vi "sub_flood-fill.vi"(10 "occupancy_map":T1, 11 "center_point":cluster{"center x":i32, "center y":i32}) -> ()   [LabVIEW 2019]
uses:
  <vilib>/Analysis/Matrix/Datatypes/RealMatrix.ctl
  <vilib>/Analysis/Matrix/NI_Matrix.lvlib
panel:
  out "sy":i32
  out "sx":i32
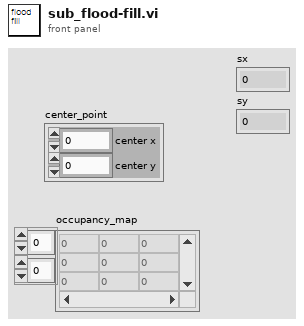
[diagram p1: front panel]
types:
  T1 = typedef "NI_Matrix.lvlib/RealMatrix.ctl" = dbl[][]
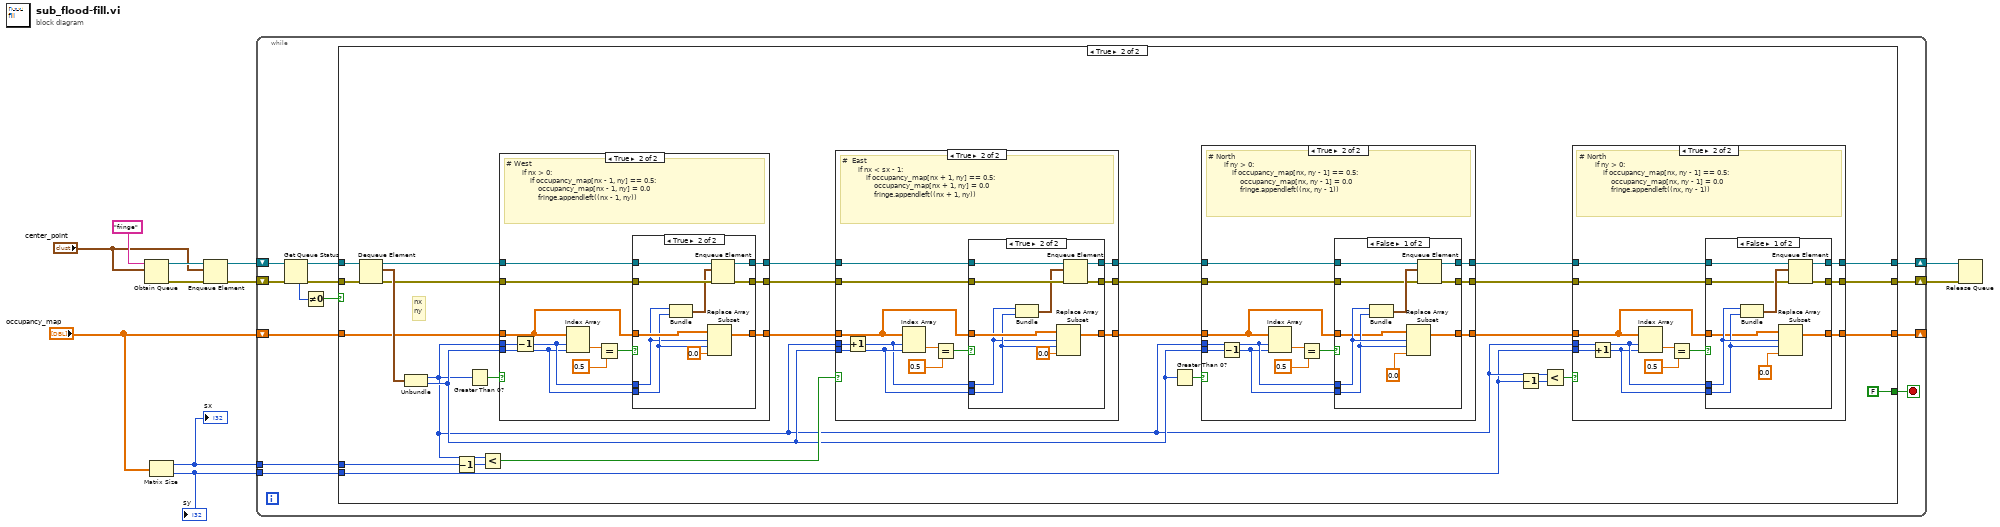
[diagram p0: block diagram]
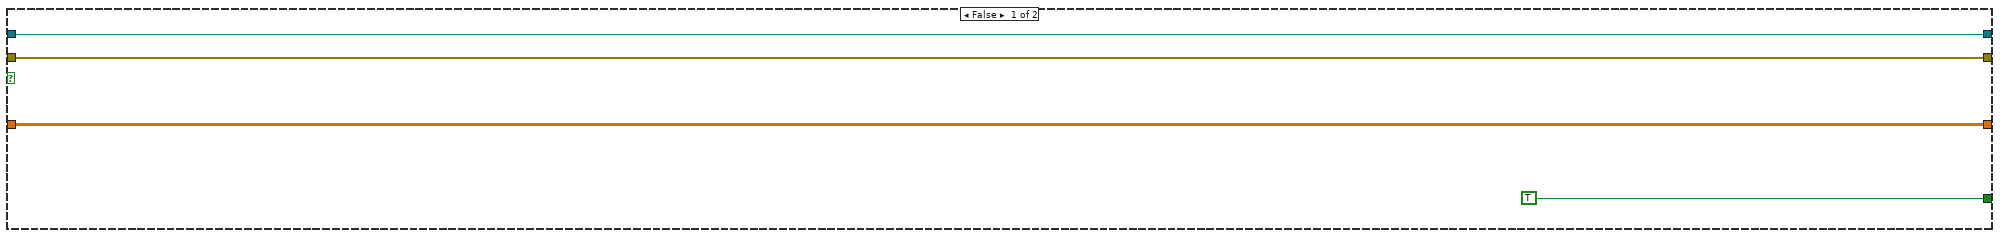
[diagram p2: hidden frame]
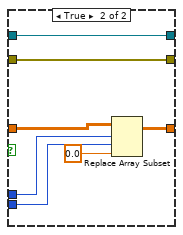
[diagram p4: hidden frame]
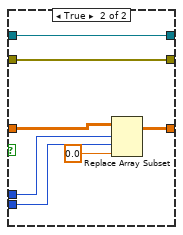
[diagram p6: hidden frame]
diagram:
  n1 = Obtain Queue(name (unnamed)="fringe", element data type="center_point") -> (queue out=w9:refnum<queue>, error out=w10:errorcluster)  [unwired: 3 in, 1 out]
  n2 = Matrix Size(0:"occupancy_map") -> (1:w2:i32, 2:w1:i32)
  "sx" <- w2
  "sy" <- w1
  n3 = Enqueue Element(queue=w9, element="center_point", error in (no error)=w10) -> (queue out=w6:refnum<queue>, error out=w7:errorcluster)  [unwired: 1 in, 1 out]
  n4 = while {
    shift-right: [w17] -> w5
    shift-left: w6 -> [w23]
    shift-right: [w16] -> w4
    shift-left: w7 -> [w24]
    shift-right: [w14] -> _
    shift-left: "occupancy_map" -> [w15]
    tunnel: w2 -> [w13]
    tunnel: w1 -> [w12]
    stop <- w20 stop-if-true
    n5 = Get Queue Status(queue=w23, error in (no error)=w24) -> (queue out=w18:refnum<queue>, error out=w19:errorcluster, # elements in queue=w22:i32)  [unwired: 1 in, 5 out]
    n6 = Not Equal To 0?(x=w22) -> (x != 0?=w21:bool)
    n7 = case shown="True" w21 {
      tunnel: [TRUE FALSE] -> w20
      tunnel: w19 -> [w26 w56]
      tunnel: w18 -> [w27 w55]
      tunnel: [w27 w36] -> w17
      tunnel: [w26 w35] -> w16
      tunnel: w15 -> [w25 w52]
      tunnel: [w25 w33] -> w14
      tunnel: w13 -> [_ w49]
      tunnel: w12 -> [_ w29]
      frame False {
      }
      frame True {
        # "nx\nny"
        n8 = Dequeue Element(queue=w55, error in (no error)=w56) -> (queue out=w44:refnum<queue>, element=w54:cluster{"center x":i32, "center y":i32}, error out=w41:errorcluster)  [unwired: 1 in, 1 out]
        n9 = Unbundle(w54) -> ("center x"=w30:i32, "center y"=w45:i32)
        n10 = Decrement(x=w49) -> (x-1=w48:i32)
        n11 = Greater Than 0?(x=w30) -> (x > 0?=w53:bool)
        n12 = Less?(x=w30, y=w48) -> (x < y?=w50:bool)
        n13 = case shown="True" w53 {
          tunnel: w52 -> [w152 w157]
          tunnel: w30 -> [_ w164]
          tunnel: w45 -> [_ w158]
          tunnel: [w152 w160] -> w51
          tunnel: w44 -> [w151 w154]
          tunnel: [w151 w153] -> w43
          tunnel: w41 -> [w150 w156]
          tunnel: [w150 w155] -> w40
          frame False {
          }
          frame True {
            # "# West\n        if nx > 0:\n            if occupancy_map[nx - 1, ny] == 0.5:\n                occupancy_map[nx - 1, ny] = 0.0\n                fringe.appendleft((nx - 1, ny))"
            n14 = Decrement(x=w164) -> (x-1=w159:i32)
            n15 = Index Array(array=w157, index (row)=w159, index (col)=w158) -> (element=w163:dbl)
            n16 = Equal?(x=w163, y=0.5) -> (x = y?=w161:bool)
            n17 = case shown="True" w161 {
              tunnel: [w167 w177] -> w160
              tunnel: w159 -> [_ w168]
              tunnel: w158 -> [_ w169]
              tunnel: w157 -> [w167 w176]
              tunnel: w156 -> [w165 w174]
              tunnel: [w165 w173] -> w155
              tunnel: w154 -> [w166 w172]
              tunnel: [w166 w171] -> w153
              frame False {
              }
              frame True {
                n18 = Bundle(w168, "center y"=w169) -> (w170:cluster{i32, "center y":i32})  [unwired: 1 in]
                n19 = Replace Array Subset(array=w176, new element=0.0 ("new element/submatrix"), index (row)=w168, index (col)=w169) -> (w177:T1)
                n20 = Enqueue Element(queue=w172, element=w170, error in (no error)=w174) -> (queue out=w171:refnum<queue>, error out=w173:errorcluster)  [unwired: 1 in, 1 out]
              }
            }
          }
        }
        n21 = case shown="True" w50 {
          tunnel: w51 -> [w124 w130]
          tunnel: w30 -> [_ w132]
          tunnel: w45 -> [_ w131]
          tunnel: [w124 w133] -> w46
          tunnel: w43 -> [w123 w128]
          tunnel: [w123 w126] -> w42
          tunnel: w40 -> [w122 w127]
          tunnel: [w122 w125] -> w39
          frame False {
          }
          frame True {
            # "#  East\n        if nx < sx - 1:\n            if occupancy_map[nx + 1, ny] == 0.5:\n                occupancy_map[nx + 1, ny] = 0.0\n                fringe.appendleft((nx + 1, ny))"
            n22 = Increment(x=w132) -> (x+1=w129:i32)
            n23 = Index Array(array=w130, index (row)=w129, index (col)=w131) -> (element=w136:dbl)
            n24 = Equal?(x=w136, y=0.5) -> (x = y?=w134:bool)
            n25 = case shown="True" w134 {
              tunnel: [w139 w149] -> w133
              tunnel: w129 -> [_ w141]
              tunnel: w131 -> [_ w142]
              tunnel: w130 -> [w139 w148]
              tunnel: w128 -> [w138 w146]
              tunnel: w127 -> [w137 w145]
              tunnel: [w138 w144] -> w126
              tunnel: [w137 w143] -> w125
              frame False {
              }
              frame True {
                n26 = Bundle(w141, "center y"=w142) -> (w140:cluster{i32, "center y":i32})  [unwired: 1 in]
                n27 = Replace Array Subset(array=w148, new element=0.0 ("new element/submatrix"), index (row)=w141, index (col)=w142) -> (w149:T1)
                n28 = Enqueue Element(queue=w146, element=w140, error in (no error)=w145) -> (queue out=w144:refnum<queue>, error out=w143:errorcluster)  [unwired: 1 in, 1 out]
              }
            }
          }
        }
        n29 = Greater Than 0?(x=w45) -> (x > 0?=w47:bool)
        n30 = case shown="True" w47 {
          tunnel: w46 -> [w92 w99]
          tunnel: w30 -> [_ w98]
          tunnel: w45 -> [_ w100]
          tunnel: [w92 w101] -> w34
          tunnel: w42 -> [w91 w96]
          tunnel: [w91 w94] -> w37
          tunnel: w39 -> [w90 w95]
          tunnel: [w90 w93] -> w38
          frame False {
          }
          frame True {
            # "# North\n        if ny > 0:\n            if occupancy_map[nx, ny - 1] == 0.5:\n                occupancy_map[nx, ny - 1] = 0.0\n                fringe.appendleft((nx, ny - 1))"
            n31 = Decrement(x=w100) -> (x-1=w97:i32)
            n32 = Index Array(array=w99, index (row)=w98, index (col)=w97) -> (element=w104:dbl)
            n33 = Equal?(x=w104, y=0.5) -> (x = y?=w102:bool)
            n34 = case shown="False" w102 {
              tunnel: [w105 w121] -> w101
              tunnel: w98 -> [w108 w120]
              tunnel: w97 -> [w107 w119]
              tunnel: w99 -> [w106 w118]
              tunnel: w96 -> [w113 w116]
              tunnel: w95 -> [w112 w115]
              tunnel: [w111 w116] -> w94
              tunnel: [w110 w115] -> w93
              frame False {
                n35 = Bundle("center x"=w108, w107) -> (w114:cluster{"center x":i32, i32})  [unwired: 1 in]
                n36 = Replace Array Subset(array=w106, new element=0.0 ("new element/submatrix"), index (row)=w108, index (col)=w107) -> (w105:T1)
                n37 = Enqueue Element(queue=w113, element=w114, error in (no error)=w112) -> (queue out=w111:refnum<queue>, error out=w110:errorcluster)  [unwired: 1 in, 1 out]
              }
              frame True {
                n38 = Replace Array Subset(array=w118, new element=0.0 ("new element/submatrix"), index (row)=w120, index (col)=w119) -> (w121:T1)
              }
            }
          }
        }
        n39 = Decrement(x=w29) -> (x-1=w31:i32)
        n40 = Less?(x=w30, y=w31) -> (x < y?=w32:bool)
        n41 = case shown="True" w32 {
          tunnel: w34 -> [w60 w67]
          tunnel: w30 -> [_ w66]
          tunnel: w29 -> [_ w68]
          tunnel: [w60 w69] -> w33
          tunnel: w37 -> [w59 w64]
          tunnel: [w59 w62] -> w36
          tunnel: w38 -> [w58 w63]
          tunnel: [w58 w61] -> w35
          frame False {
          }
          frame True {
            # "# North\n        if ny > 0:\n            if occupancy_map[nx, ny - 1] == 0.5:\n                occupancy_map[nx, ny - 1] = 0.0\n                fringe.appendleft((nx, ny - 1))"
            n42 = Increment(x=w68) -> (x+1=w65:i32)
            n43 = Index Array(array=w67, index (row)=w66, index (col)=w65) -> (element=w72:dbl)
            n44 = Equal?(x=w72, y=0.5) -> (x = y?=w70:bool)
            n45 = case shown="False" w70 {
              tunnel: [w73 w89] -> w69
              tunnel: w66 -> [w76 w88]
              tunnel: w65 -> [w75 w87]
              tunnel: w67 -> [w74 w86]
              tunnel: w64 -> [w77 w84]
              tunnel: w63 -> [w78 w83]
              tunnel: [w81 w84] -> w62
              tunnel: [w80 w83] -> w61
              frame False {
                n46 = Bundle("center x"=w76, w75) -> (w82:cluster{"center x":i32, i32})  [unwired: 1 in]
                n47 = Replace Array Subset(array=w74, new element=0.0 ("new element/submatrix"), index (row)=w76, index (col)=w75) -> (w73:T1)
                n48 = Enqueue Element(queue=w77, element=w82, error in (no error)=w78) -> (queue out=w81:refnum<queue>, error out=w80:errorcluster)  [unwired: 1 in, 1 out]
              }
              frame True {
                n49 = Replace Array Subset(array=w86, new element=0.0 ("new element/submatrix"), index (row)=w88, index (col)=w87) -> (w89:T1)
              }
            }
          }
        }
      }
    }
  }
  n50 = Release Queue(queue=w5, error in (no error)=w4) -> ()  [unwired: 1 in, 3 out]
